vi "Test.vi"   [LabVIEW 2012]
uses:
  <vilib>/Distrio/Murmex/Murmex/Murmex.lvclass
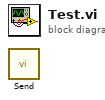
[diagram p0: block diagram]
diagram:
  n1 = call <vilib>:"Send.vi"() -> ()  [unwired: 10 in, 2 out]
